vi "Round Timestamp to Second.vi"(1 "Time Stamp (now)":timestamp) -> (0 "Time Stamp":timestamp)   [LabVIEW 2011]
doc: "Rounds Timestamp to the nearest second.\n\nReturns current time if input is unwired.\n\nVersion 1.0 - 03/07/2013\n\nPhaeron, Inc.\nwww.phaeron.com\ninfo@phaeron.com"
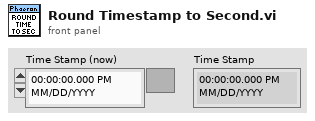
[diagram p1: front panel]
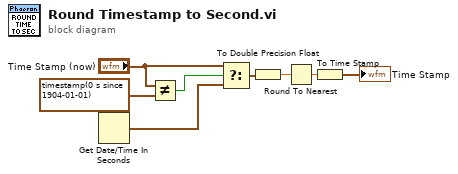
[diagram p0: block diagram]
diagram:
  n1 = Get Date/Time In Seconds() -> (seconds since 1Jan1904=w1:timestamp)
  n2 = Not Equal?(x="Time Stamp (now)", y=timestamp(0 s since 1904-01-01) ("Time Stamp")) -> (x != y?=w4:bool)
  n3 = Select(t="Time Stamp (now)", s=w4, f=w1) -> (s? t:f=w2:timestamp)
  n4 = To Double Precision Float(number=w2) -> (double precision float=w6:dbl)
  n5 = Round To Nearest(number=w6) -> (nearest integer value=w8:dbl)
  n6 = To Time Stamp(1:w8) -> (0:→"Time Stamp":timestamp)
